vi "趋势项消除.vi"(1 "采样频率":dbl, 2 "数组":dbl[](array[numeric])) -> (0 "数组 2":dbl[](array[numeric]))   [LabVIEW 2014]
uses:
  <vilib>/Analysis/4window.llb/Exponential Window (DBL).vi
  <vilib>/Analysis/NI_AALPro.lvlib
panel:
  out "b1":dbl
  out "b0":dbl
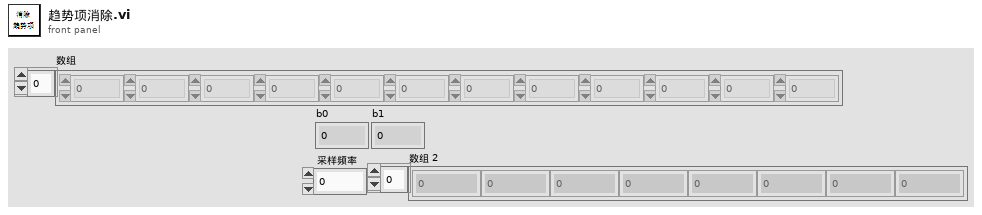
[diagram p1: front panel]
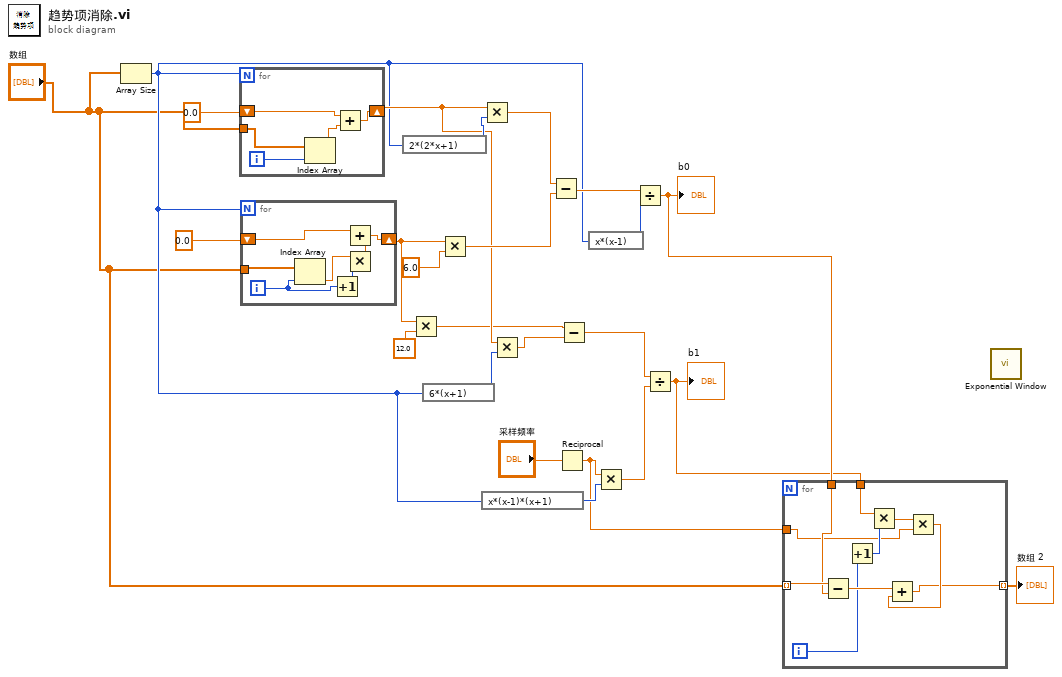
[diagram p0: block diagram]
diagram:
  n1 = Array Size(array="数组") -> (size(s)=w9:i32)
  n2 = for {
    N: w9 -> [_]
    shift-right: [w28] -> w13
    shift-left: 0.0 -> [w29]
    tunnel: "数组" -> [w27]
    i -> [w25]
    n3 = Index Array(array=w27, index=w25) -> (element=w26:dbl)
    n4 = Add(x=w29, y=w26) -> (x+y=w28:dbl)
  }
  n5 = for {
    N: w9 -> [_]
    shift-right: [w30] -> w16
    shift-left: 0.0 -> [w31]
    tunnel: "数组" -> [w36]
    i -> [w34]
    n6 = Index Array(array=w36, index=w34) -> (element=w35:dbl)
    n7 = Increment(x=w34) -> (x+1=w33:i32)
    n8 = Multiply(x=w35, y=w33) -> (x*y=w32:dbl)
    n9 = Add(x=w31, y=w32) -> (x+y=w30:dbl)
  }
  n10 = expression code="2*(2*x+1)"(w9) -> (w23:i32)
  n11 = Multiply(x=w16, y=12.0) -> (x*y=w12:dbl)
  n12 = expression code="6*(x+1)"(w9) -> (w14:i32)
  n13 = Multiply(x=w16, y=6.0) -> (x*y=w19:dbl)
  n14 = Multiply(x=w13, y=w23) -> (x*y=w20:dbl)
  n15 = expression code="x*(x-1)*(x+1)"(w9) -> (w8:i32)
  n16 = Multiply(x=w13, y=w14) -> (x*y=w11:dbl)
  n17 = Subtract(x=w20, y=w19) -> (x-y=w18:dbl)
  n18 = Reciprocal(x="采样频率") -> (1/x=w2:dbl)
  n19 = Subtract(x=w12, y=w11) -> (x-y=w7:dbl)
  n20 = expression code="x*(x-1)"(w9) -> (w17:i32)
  n21 = Multiply(x=w2, y=w8) -> (x*y=w6:dbl)
  n22 = Divide(x=w18, y=w17) -> (x/y=w4:dbl)
  "b0" <- w4
  n23 = Divide(x=w7, y=w6) -> (x/y=w3:dbl)
  "b1" <- w3
  n24 = for {
    tunnel: "数组" -> [w46] mode=indexing
    tunnel: w4 -> [w45]
    tunnel: w3 -> [w43]
    tunnel: w2 -> [w39]
    tunnel: [w37] -> w1 mode=indexing
    i -> [w42]
    n25 = Subtract(x=w46, y=w45) -> (x-y=w44:dbl)
    n26 = Increment(x=w42) -> (x+1=w41:i32)
    n27 = Multiply(x=w43, y=w41) -> (x*y=w40:dbl)
    n28 = Multiply(x=w40, y=w39) -> (x*y=w38:dbl)
    n29 = Add(x=w44, y=w38) -> (x+y=w37:dbl)
  }
  "数组 2" <- w1
  n30 = call-poly <vilib>:"Exponential Window.vi"() -> ()  [unwired: 2 in, 2 out]
